vi "udp_test.vi"() -> ()   [LabVIEW 2020]
uses:
  LabVIEW/Aerial_Ladder_Truck/RealTime/control/sensor_data.ctl
panel:
  out "x-y":u32
  out "Waveform Chart":dbl(graph)
  out "net address":u32
  out "data_out":dbl[](array[numeric])
  out "sensor_data":T1
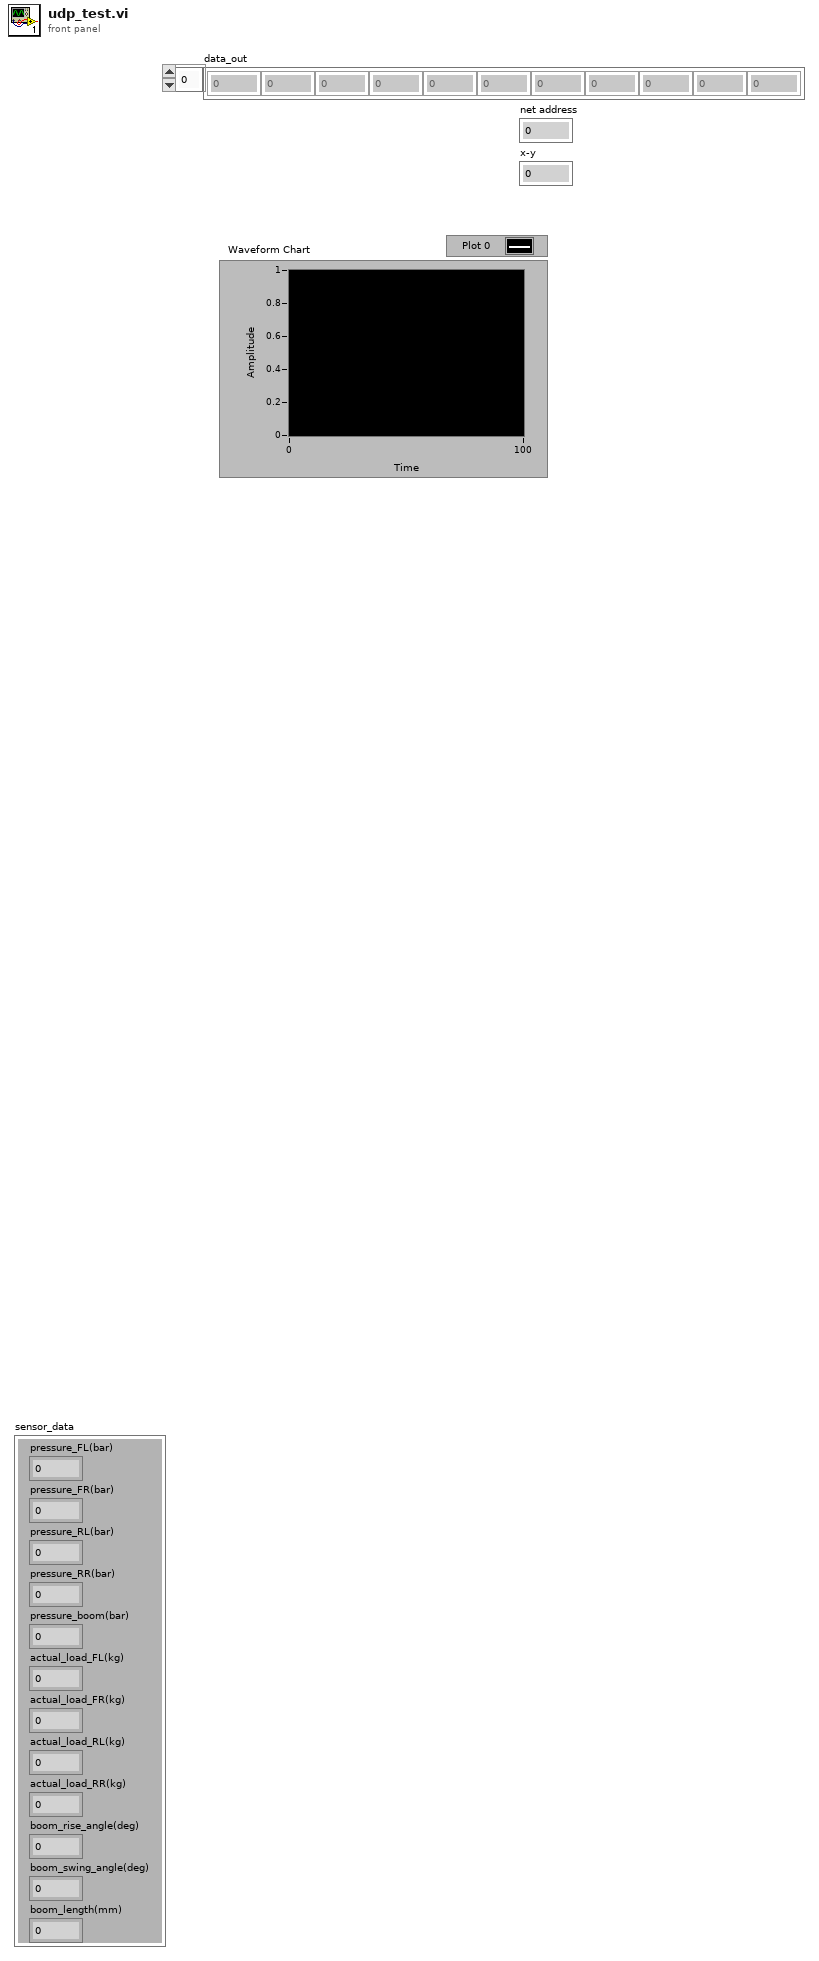
[diagram p1: front panel]
types:
  T1 = typedef "sensor_data.ctl" = cluster{"pressure_FL(bar)":dbl, "pressure_FR(bar)":dbl, "pressure_RL(bar)":dbl, "pressure_RR(bar)":dbl, "pressure_boom(bar)":dbl, "actual_load_FL(kg)":dbl, "actual_load_FR(kg)":dbl, "actual_load_RL(kg)":dbl, "actual_load_RR(kg)":dbl, "boom_rise_angle(deg)":dbl, "boom_swing_angle(deg)":dbl, "boom_length(mm)":dbl}
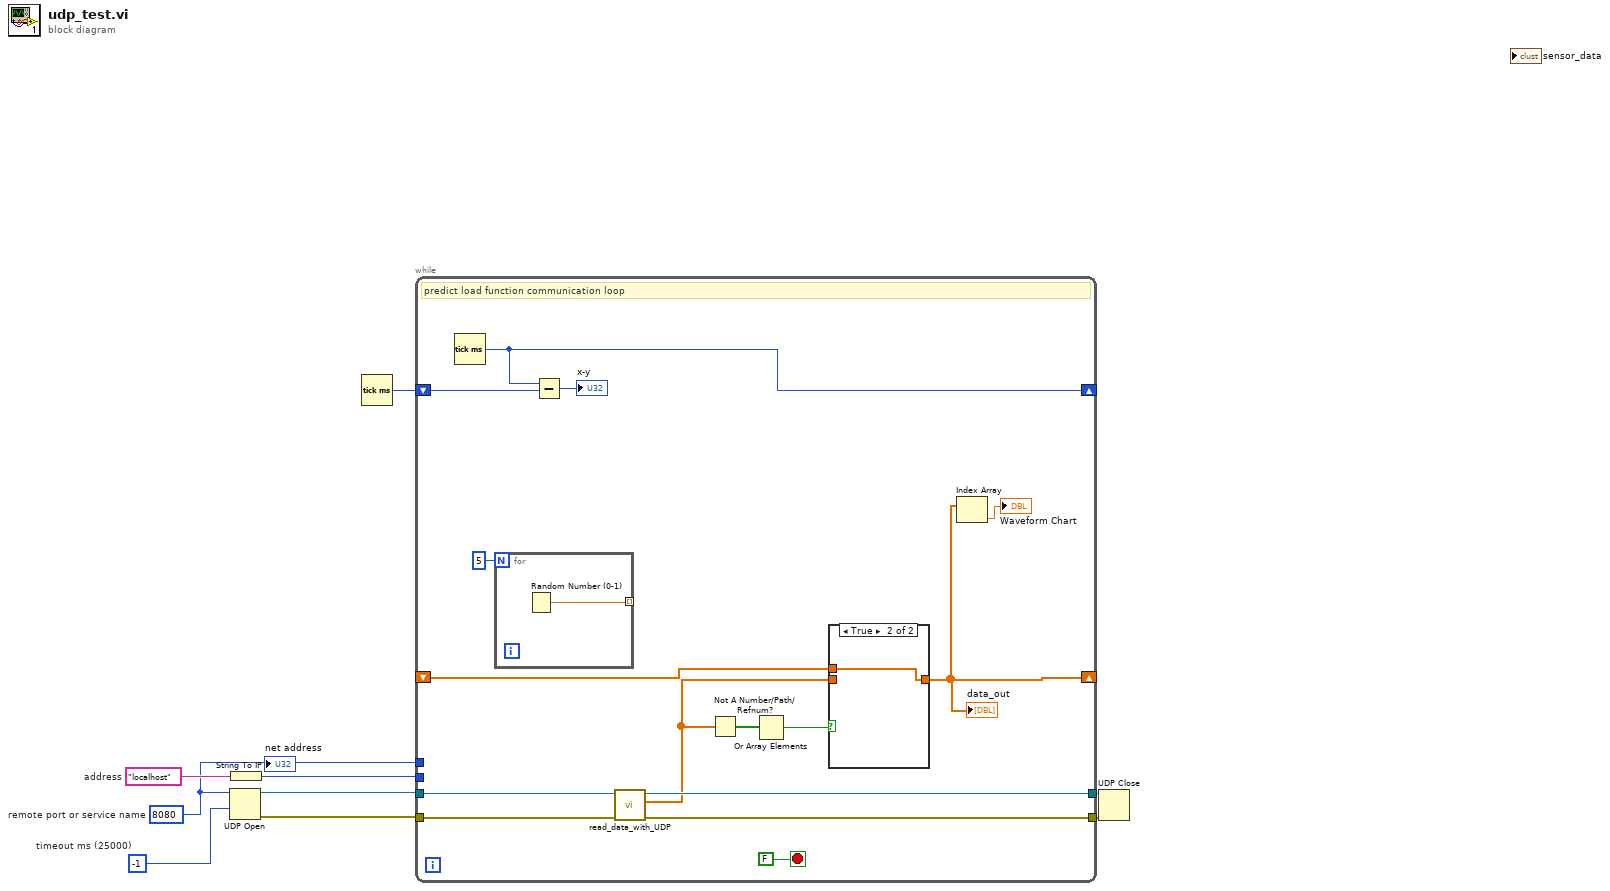
[diagram p0: block diagram]
diagram:
  w3 = -1  # timeout ms (25000)
  w9 = "localhost"  # address
  w7 = u16 8080  # remote port or service name
  n1 = UDP Open(9:w3, 11:w7) -> (port=w8:refnum<k16>, 0:w6:errorcluster)  [unwired: 3 in, 1 out]
  n2 = String To IP(1:w9) -> (0:w2:u32)
  n3 = Tick Count (ms)() -> (millisecond timer value=w1:u32)
  n4 = while {
    tunnel: w6 -> [w21]
    tunnel: w8 -> [w22]
    tunnel: w2 -> [_]
    tunnel: w7 -> [_]
    tunnel: [w20] -> w5
    tunnel: [w19] -> w4
    shift-right: [w14] -> _
    shift-left: _ -> [w15]
    shift-right: [w12] -> _
    shift-left: w1 -> [w11]
    stop <- FALSE stop-if-true
    # "predict load function communication loop"
    n5 = Tick Count (ms)() -> (millisecond timer value=w12:u32)
    n6 = for {
      N: 5 -> [_]
      tunnel: [w27] -> _ mode=indexing
      n7 = Random Number (0-1)() -> (number: 0 to 1=w27:dbl)
    }
    n8 = Subtract(x=w12, y=w11) -> (x-y=→"x-y":u32)
    n9 = call "read_data_with_UDP.vi"("error_in"=w21, "udp_ref_in"=w22) -> ("error_out"=w19:errorcluster, "data_out"=w16:dbl[], "udp_ref_out"=w20:refnum<k16>)  [unwired: 7 in]
    n10 = Not A Number/Path/Refnum?(number/path/refnum=w16) -> (NaN/Path/Refnum?=w18:bool[])
    n11 = Or Array Elements(Boolean array=w18) -> (logical OR=w17:bool)
    n12 = case shown="True" w17 {
      tunnel: [w25 w26] -> w14
      tunnel: w16 -> [w25 _]
      tunnel: w15 -> [_ w26]
      frame False {
      }
      frame True {
      }
    }
    "data_out" <- w14
    n13 = Index Array(array=w14) -> (element=→"Waveform Chart":dbl)  [unwired: 1 in]
  }
  n14 = UDP Close(connection ID=w5, 8:w4) -> ()  [unwired: 2 out]
